vi "Get Configuration File Path.vi"(8 "error in (no error)":errorcluster) -> (0 "error out":errorcluster, 3 "XML File Path":path)   [LabVIEW 2014]
doc: "Get the path to the Settings XML file. This is done using the Application Directory function. For more information on how Application Directory calculates its path, right-click the function and choose Help."
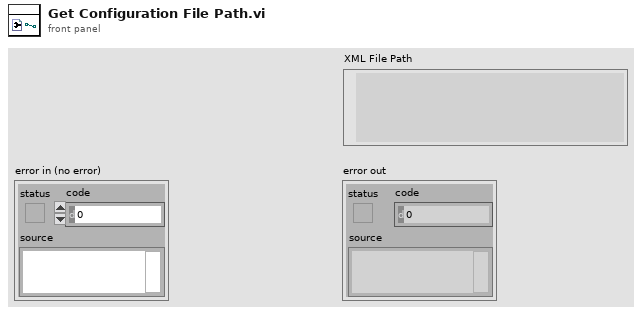
[diagram p1: front panel]
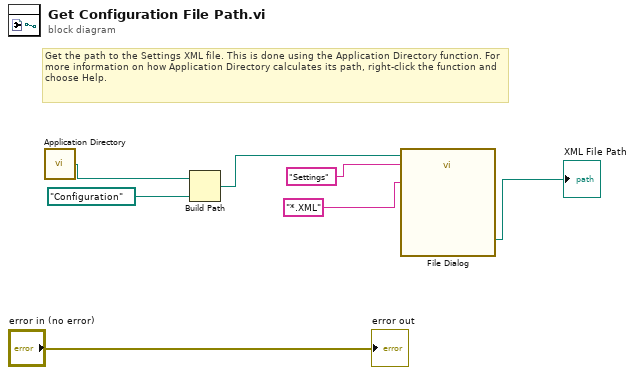
[diagram p0: block diagram]
diagram:
  # "Get the path to the Settings XML file. This is done using the Application Directory function. For more information on how Application Directory calculates its path, right-click the function and choose Help."
  n1 = call <vilib>:"Application Directory.vi"() -> ("Application Directory"=w2:path)
  n2 = Build Path(base path=w2, name or relative path=path "Configuration") -> (appended path=w1:path)
  n3 = call "File Dialog"("start path"=w1, "default name"="Settings", "pattern (all files)"="*.XML") -> ("selected path"=→"XML File Path":path)  [unwired: 9 in, 3 out]
  "error out" <- "error in (no error)"
